vi "ATF Storage-DI_Scale.vi"(8 "error in (no error)":errorcluster, 10 "DI":T1(array[cluster]), 11 "Refnum in":refnum<k21>) -> (0 "error out":errorcluster, 3 "Refnum out":refnum<k21>)   [LabVIEW 2022 SP3]
uses:
  <vilib>/DAQmx/create/channels.llb/DAQmx Create Channel (DI-Digital Input).vi
  <resource>/objmgr/daqmx.rc
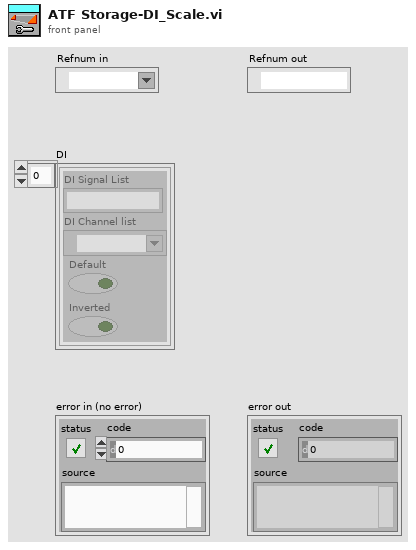
[diagram p1: front panel]
types:
  T1 = cluster{"DI Signal List":string, "DI Channel list":tag, "Default":bool, "Inverted":bool}[]
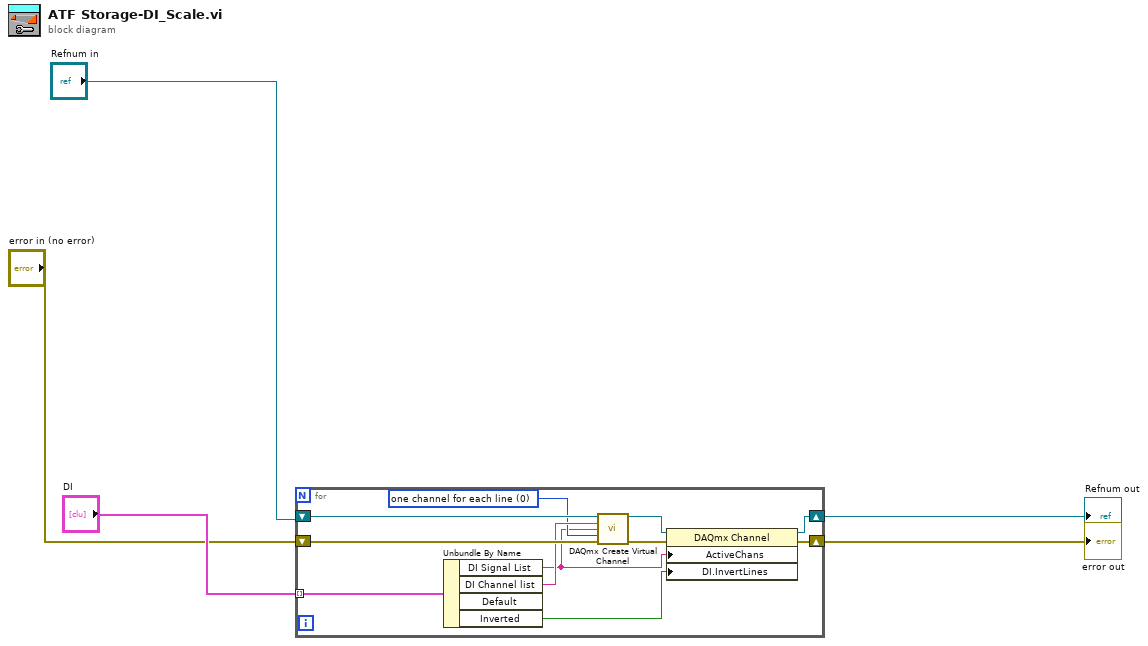
[diagram p0: block diagram]
diagram:
  n1 = for {
    tunnel: "DI" -> [w16] mode=indexing
    shift-right: [w9] -> w1
    shift-left: "Refnum in" -> [w15]
    shift-right: [w8] -> w2
    shift-left: "error in (no error)" -> [w14]
    w12 = 0 items=["one channel for each line", "one channel for all lines"] ("line grouping")
    n2 = Unbundle By Name(w16) -> ("DI Signal List"=w7:string, "DI Channel list"=w13:tag, "Inverted"=w6:bool)  [unwired: 1 out]
    n3 = call-poly <vilib>:"DAQmx Create Virtual Channel.vi"("task in"=w15, "lines"=w13, "name to assign"=w7, "line grouping"=w12, "error in"=w14) -> ("task out"=w11:refnum<k21>, "error out"=w10:errorcluster)  [unwired: 9 in]
    n4 = property on="Property Node" class="DAQmx Channel"(reference=w11, error in=w10, "ActiveChans"=w7, "DI.InvertLines"=w6) -> (reference out=w9:refnum<k21>, error out=w8:errorcluster)
  }
  "error out" <- w2
  "Refnum out" <- w1
